vi "NoParent_TreeHasTagWithPrefixAndName.vi"() -> (0 "error out":errorcluster)   [LabVIEW 2017, in "ResultTree.Tests.lvlib" / "AddTestSuite.lvlib"]
uses:
  AddTestSuite.lvlib
  2a6c7ef5-d8ea-4de4-ba7d-c6663dbf2225.vi
  Constraint/IsEqual/Create.vi
  Constraint/IsEqual/IsEqual.lvclass
  ResultTree/ResultTree.lvclass
panel:
  in  "Tree":string(tree)
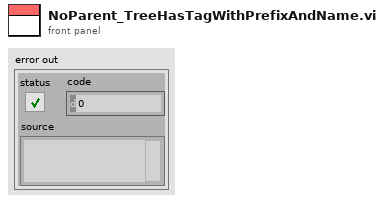
[diagram p1: front panel]
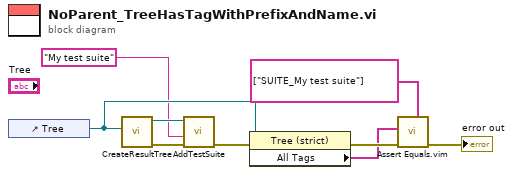
[diagram p0: block diagram]
diagram:
  n1 = control-ref of="Tree"() -> (w8:refnum<vi>)
  n2 = call "CreateResultTree.vi"("Tree Refnum"=w8) -> ("error out"=w7:errorcluster, "ResultTree out"=w5:refnum<class "ResultTree.lvclass">)  [unwired: 9 in]
  n3 = call "AddTestSuite.vi"("error in (no error)"=w7, "Name"="My test suite", "ResultTree in"=w5) -> ("error out"=w6:errorcluster)  [unwired: 6 in, 2 out]
  n4 = property class="Tree (strict)"(reference=w8, error in=w6) -> (error out=w4:errorcluster, "All Tags"=w3:string[])  [unwired: 1 out]
  n5 = call "Assert Equals.vim"("Expected"=string[] ["SUITE_My test suite"] ("All Tags"), "error in (no error)"=w4, "Actual"=w3) -> ("error out"=→"error out":errorcluster)  [unwired: 8 in]
